vi "LNLS Control Encode FOFBC.vi"(8 "error in (no error)":errorcluster, 11 "PFOFBC Data":T1={"Status"=0, "Operation Mode"=enum."Manual Mode", "PID Horizontal Gain"=0.0, "PID Vertical Gain"=0.0, "PID Horizontal Integral Time"=0.0, "PID Vertical Integral Time"=0.0, "PID Horizontal Derivative Time"=0.0, "PID Vertical Derivative Time"=0.0, "Fast Command Enabled"=FALSE, "RMS Horizontal Distortion"=0.0, "RMS Vertical Distortion"=0.0, "Timestamp"=0.0}) -> (0 "error out":errorcluster, 2 "command body":string)   [LabVIEW 2011, in "LNLS Control VIs.lvlib"]
uses:
  LNLS Control VIs.lvlib
  Types Definitions/Type Control FOFB Configuration Out.ctl
  Types Definitions/Type Operation Mode State.ctl
  Type Definitions.lvlib
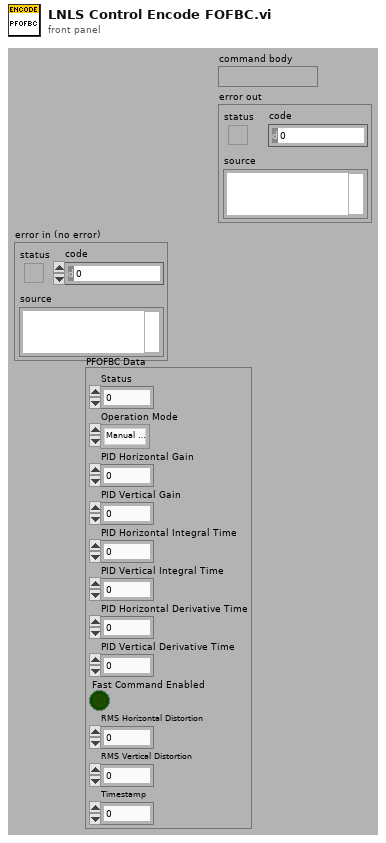
[diagram p1: front panel]
types:
  T1 = typedef "Type Definitions.lvlib/Type Control FOFB Configuration Out.ctl" = cluster{"Status":u16, "Operation Mode":T2, "PID Horizontal Gain":sgl, "PID Vertical Gain":sgl, "PID Horizontal Integral Time":sgl, "PID Vertical Integral Time":sgl, "PID Horizontal Derivative Time":sgl, "PID Vertical Derivative Time":sgl, "Fast Command Enabled":bool, "RMS Horizontal Distortion":dbl, "RMS Vertical Distortion":dbl, "Timestamp":dbl}
  T2 = typedef "Type Definitions.lvlib/Type Operation Mode State.ctl" = enum8{"Idle Mode", "Manual Mode", "FOFB Mode", "RMM Mode"}
  T3 = enum16{"big-endian, network order", "native, host order", "little-endian"}
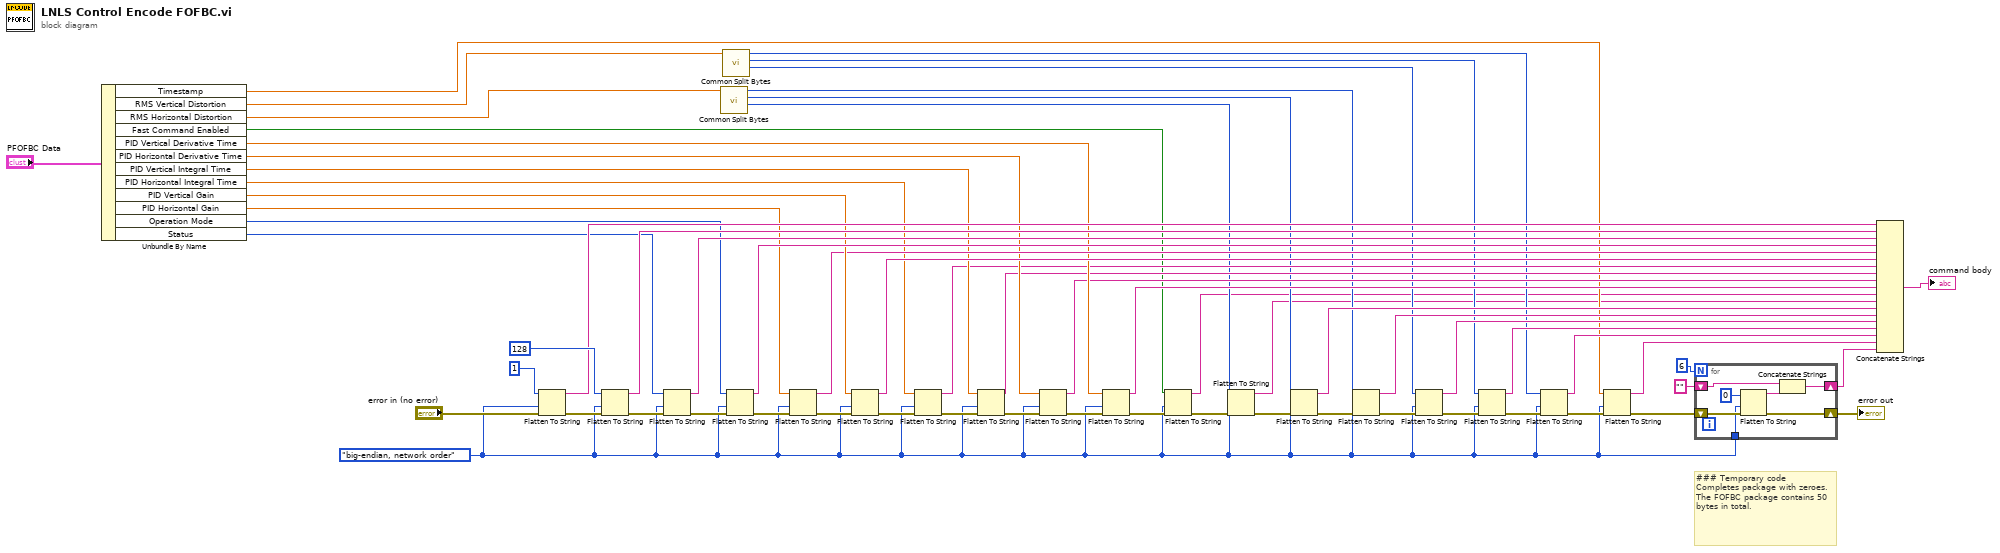
[diagram p0: block diagram]
diagram:
  w4 = T3."big-endian, network order" ("byte order (0:big-endian, network order)")
  # "### Temporary code\nCompletes package with zeroes. The FOFBC package contains 50 bytes in total."
  n1 = Unbundle By Name("PFOFBC Data") -> ("Timestamp"=w8:dbl, "RMS Vertical Distortion"=w19:dbl, "RMS Horizontal Distortion"=w15:dbl, "Fast Command Enabled"=w5:bool, "PID Vertical Derivative Time"=w39:sgl, "PID Horizontal Derivative Time"=w40:sgl, "PID Vertical Integral Time"=w41:sgl, "PID Horizontal Integral Time"=w42:sgl, "PID Vertical Gain"=w47:sgl, "PID Horizontal Gain"=w48:sgl, "Operation Mode"=w44:T2, "Status"=w43:u16)
  n2 = Flatten To String(anything=u8 1 ("priority"), byte order (0:big-endian, network order)=w4, error in (no error)="error in (no error)") -> (data string=w56:string, error out=w58:errorcluster)  [unwired: 1 in, 1 out]
  n3 = Flatten To String(anything=u8 128 ("flag"), byte order (0:big-endian, network order)=w4, error in (no error)=w58) -> (data string=w57:string, error out=w52:errorcluster)  [unwired: 1 in, 1 out]
  n4 = Flatten To String(anything=w43, byte order (0:big-endian, network order)=w4, error in (no error)=w52) -> (data string=w50:string, error out=w63:errorcluster)  [unwired: 1 in, 1 out]
  n5 = call "Common Split Bytes.vi"("Double"=w15) -> ("Most Significant Byte"=w12:u8, "Intermediate Byte"=w13:u8, "Less Significant Byte"=w14:u8)  [unwired: 8 in]
  n6 = call "Common Split Bytes.vi"("Double"=w19) -> ("Most Significant Byte"=w16:u8, "Intermediate Byte"=w17:u8, "Less Significant Byte"=w18:u8)  [unwired: 8 in]
  n7 = Flatten To String(anything=w44, byte order (0:big-endian, network order)=w4, error in (no error)=w63) -> (data string=w49:string, error out=w51:errorcluster)  [unwired: 1 in, 1 out]
  n8 = Flatten To String(anything=w48, byte order (0:big-endian, network order)=w4, error in (no error)=w51) -> (data string=w46:string, error out=w62:errorcluster)  [unwired: 1 in, 1 out]
  n9 = Flatten To String(anything=w47, byte order (0:big-endian, network order)=w4, error in (no error)=w62) -> (data string=w45:string, error out=w38:errorcluster)  [unwired: 1 in, 1 out]
  n10 = Flatten To String(anything=w42, byte order (0:big-endian, network order)=w4, error in (no error)=w38) -> (data string=w29:string, error out=w37:errorcluster)  [unwired: 1 in, 1 out]
  n11 = Flatten To String(anything=w41, byte order (0:big-endian, network order)=w4, error in (no error)=w37) -> (data string=w28:string, error out=w36:errorcluster)  [unwired: 1 in, 1 out]
  n12 = Flatten To String(anything=w40, byte order (0:big-endian, network order)=w4, error in (no error)=w36) -> (data string=w27:string, error out=w35:errorcluster)  [unwired: 1 in, 1 out]
  n13 = Flatten To String(anything=w39, byte order (0:big-endian, network order)=w4, error in (no error)=w35) -> (data string=w26:string, error out=w7:errorcluster)  [unwired: 1 in, 1 out]
  n14 = Flatten To String(anything=w5, byte order (0:big-endian, network order)=w4, error in (no error)=w7) -> (data string=w2:string, error out=w6:errorcluster)  [unwired: 1 in, 1 out]
  n15 = Flatten To String(anything=w12, byte order (0:big-endian, network order)=w4, error in (no error)=w6) -> (data string=w3:string, error out=w34:errorcluster)  [unwired: 1 in, 1 out]
  n16 = Flatten To String(anything=w13, byte order (0:big-endian, network order)=w4, error in (no error)=w34) -> (data string=w25:string, error out=w33:errorcluster)  [unwired: 1 in, 1 out]
  n17 = Flatten To String(anything=w14, byte order (0:big-endian, network order)=w4, error in (no error)=w33) -> (data string=w24:string, error out=w32:errorcluster)  [unwired: 1 in, 1 out]
  n18 = Flatten To String(anything=w16, byte order (0:big-endian, network order)=w4, error in (no error)=w32) -> (data string=w23:string, error out=w31:errorcluster)  [unwired: 1 in, 1 out]
  n19 = Flatten To String(anything=w17, byte order (0:big-endian, network order)=w4, error in (no error)=w31) -> (data string=w22:string, error out=w30:errorcluster)  [unwired: 1 in, 1 out]
  n20 = Flatten To String(anything=w18, byte order (0:big-endian, network order)=w4, error in (no error)=w30) -> (data string=w21:string, error out=w10:errorcluster)  [unwired: 1 in, 1 out]
  n21 = Flatten To String(anything=w8, byte order (0:big-endian, network order)=w4, error in (no error)=w10) -> (data string=w1:string, error out=w9:errorcluster)  [unwired: 1 in, 1 out]
  n22 = for {
    N: 6 -> [_]
    shift-right: [w70] -> w55
    shift-left: w9 -> [w71]
    shift-right: [w68] -> w20
    shift-left: "" -> [w67]
    tunnel: w4 -> [w65]
    n23 = Flatten To String(anything=u8 0 ("Correction Period (usec)"), byte order (0:big-endian, network order)=w65, error in (no error)=w71) -> (data string=w69:string, error out=w70:errorcluster)  [unwired: 1 in, 1 out]
    n24 = Concatenate Strings(w67, w69) -> (w68:string)
  }
  "error out" <- w55
  n25 = Concatenate Strings(w56, w57, w50, w49, w46, w45, w29, w28, w27, w26, w2, w3, w25, w24, w23, w22, w21, w1, w20) -> (→"command body":string)
